vi "BN_outputLayer.vi"(7 "Learning rate":fxp<+/-,32,8>, 8 "Out_outX":fxp<+/-,32,8>[](array[numeric]), 9 "Out_hx":fxp<+/-,32,8>[](array[numeric]), 10 "Target_outX":fxp<+/-,32,8>[](array[numeric]), 11 "Weights_outX_IN":fxp<+/-,32,8>[][](array[numeric])) -> (1 "Weights_outX_OUT":fxp<+/-,32,8>[][](array[numeric]))   [LabVIEW 2016]
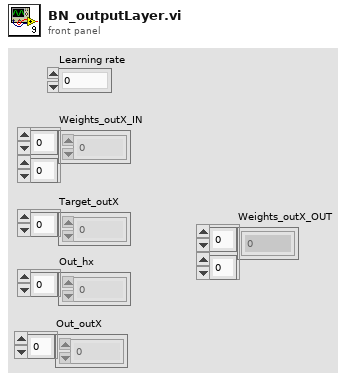
[diagram p1: front panel]
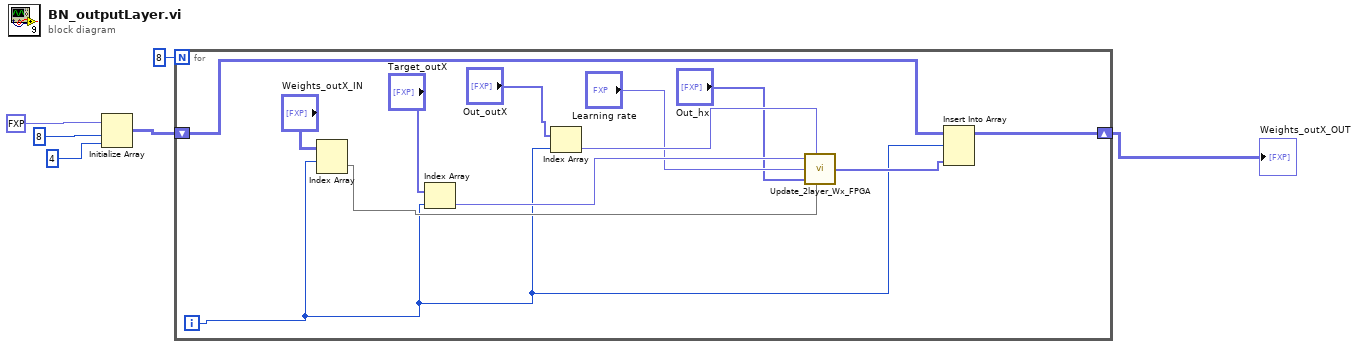
[diagram p0: block diagram]
diagram:
  n1 = Initialize Array(fxp<+,32,8> 0.0 ("element"), 8 ("dimension size"), 4 ("dimension size")) -> (w6:fxp<+,32,8>[][])
  n2 = for {
    N: 8 -> [_]
    shift-right: [w8] -> w4
    shift-left: w6 -> [w7]
    i -> [w9]
    n3 = Index Array(array="Weights_outX_IN", index (row)=w9) -> (element=w11:fxp<+/-,32,8>[])  [unwired: 1 in]
    n4 = Index Array(array="Target_outX", index=w9) -> (element=w14:fxp<+/-,32,8>)
    n5 = Index Array(array="Out_outX", index=w9) -> (element=w15:fxp<+/-,32,8>)
    n6 = call "Update_2layer_Wx_FPGA.vi"("Target_OutX"=w14, "2layer_OutX"=w15, "Learning rate"="Learning rate", "Array_Out_hx"="Out_hx", "Weights_2layer"=w11) -> ("Weights_2layer_updated"=w10:fxp<+/-,32,8>[])
    n7 = Insert Into Array(array=w7, index (row)=w9, new element=w10) -> (w8:fxp<+,32,8>[][])  [unwired: 1 in]
  }
  "Weights_outX_OUT" <- w4
